vi "Global Vars.vi"() -> ()   [LabVIEW 2015]
panel:
  in  "Soleniod":string="Four Motors"
  in  "Indexer":string="Joystick 1"
  in  "Shooter":string="Joystick 1"
  in  "Gunner":string="Joystick 1"
  in  "Driver":string="Joystick 0"
  in  "Four Motors":string="Four Motors"
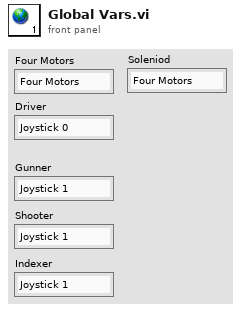
[diagram p1: front panel]
diagram:
